vi "CMI ADS127L21 - Config EXTOUT.vi"(7 "Polarity":T1, 8 "error in (no error)":errorcluster, 9 "Divisor (1)":i32=1 min=1 step=1, 10 "Mode":T2, 11 "session in":T3 {"channels"."Channel" min=1 max=8 step=1}) -> (0 "error out":errorcluster, 3 "session out":T3 {"channels"."Channel" min=1 max=8 step=1})   [LabVIEW 2020]
doc: "Config EXTOUT programmable output."
uses:
  CMI ADS127L21 - Session.ctl
  CMI ADS127L21 - Record Channel.ctl
  CMI ADS127L21 - Input Range.ctl
  CMI ADS127L21 - Input Mode.ctl
  CMI ADS127L21 - Input Impedance.ctl
  CMI ADS127L21 - EXTOUT Mode.ctl
  CMI ADS127L21 - EXTOUT Polarity.ctl
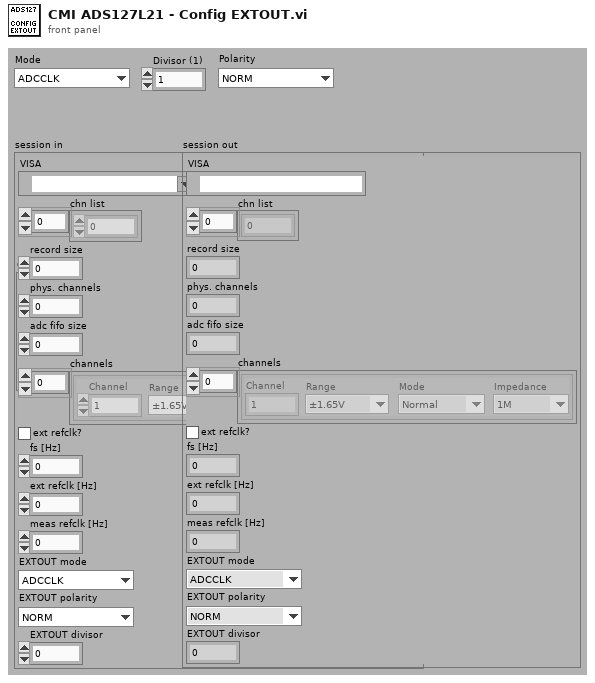
[diagram p1: front panel]
types:
  T1 = typedef "CMI ADS127L21 - EXTOUT Polarity.ctl" = enum16{"NORM", "INV"}
  T2 = typedef "CMI ADS127L21 - EXTOUT Mode.ctl" = enum16{"ADCCLK", "REFCLK", "SMPLCLK", "FIRST"}
  T3 = typedef "CMI ADS127L21 - Session.ctl" = cluster{"VISA":refnum<visa-resource-name>, "chn list":i32[], "record size":i32, "phys. channels":i32, "adc fifo size":i32, "channels":T4[], "ext refclk?":bool, "fs [Hz]":dbl, "ext refclk [Hz]":dbl, "meas refclk [Hz]":dbl, "EXTOUT mode":T2, "EXTOUT polarity":T1, "EXTOUT divisor":i32}
  T4 = typedef "CMI ADS127L21 - Record Channel.ctl" = cluster{"Range":T5, "Channel":i32, "Mode":T6, "Impedance":T7}
  T5 = typedef "CMI ADS127L21 - Input Range.ctl" = enum16{"±1.65V", "±2V"}
  T6 = typedef "CMI ADS127L21 - Input Mode.ctl" = enum16{"Normal", "Inverted", "GND"}
  T7 = typedef "CMI ADS127L21 - Input Impedance.ctl" = enum16{"1M", "1k5"}
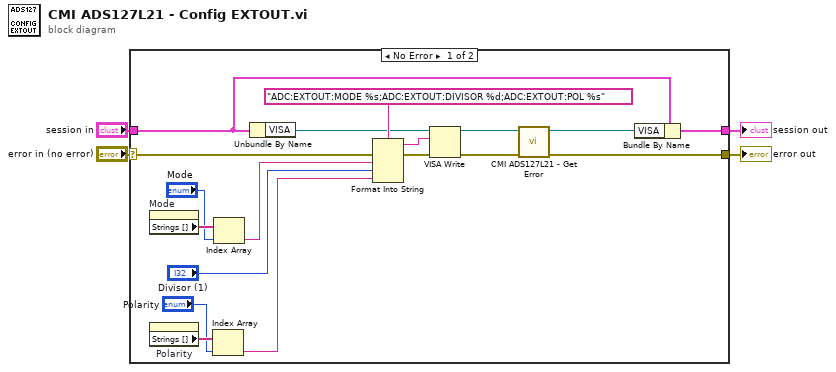
[diagram p0: block diagram]
diagram:
  n1 = case shown="No Error" "error in (no error)" {
    selector: "error in (no error)" -> [w17 w24]
    tunnel: "session in" -> [w14 w23]
    tunnel: [w15 w23] -> w3
    tunnel: [w6 w24] -> w2
    frame No Error {
      n2 = property on="Mode" class="Enum (strict)"() -> ("Strings []"=w13:string[])  [unwired: 2 in, 2 out]
      n3 = property on="Polarity" class="Enum (strict)"() -> ("Strings []"=w9:string[])  [unwired: 2 in, 2 out]
      n4 = Index Array(array=w9, index="Polarity") -> (element=w7:string)
      n5 = Index Array(array=w13, index="Mode") -> (element=w11:string)
      n6 = Unbundle By Name(w14) -> ("VISA"=w16:refnum<visa-resource-name>)
      n7 = Format Into String(format string="ADC:EXTOUT:MODE %s;ADC:EXTOUT:DIVISOR %d;ADC:EXTOUT:POL %s", error in=w17, w11, "Divisor (1)", w7) -> (resulting string=w18:string, error out=w21:errorcluster)  [unwired: 1 in]
      n8 = VISA Write(VISA resource name=w16, write buffer=w18, error in (no error)=w21) -> (VISA resource name out=w19:refnum<visa-resource-name>, error out=w20:errorcluster)  [unwired: 1 out]
      n9 = call "CMI ADS127L21 - Get Error.vi"("error in (no error)"=w20, "VISA in"=w19) -> ("error out"=w6:errorcluster, "VISA out"=w5:refnum<visa-resource-name>)  [unwired: 8 in]
      n10 = Bundle By Name(cluster=w14, "VISA"=w5) -> (w15:T3)
    }
    frame Error {
    }
  }
  "error out" <- w2
  "session out" <- w3
